vi "Move Parent FP to 0.vi"(8 "error in":errorcluster) -> (0 "error out":errorcluster)   [LabVIEW 2011]
doc: "Moves parent window to 0,0\n\n\nVersion 1.0 - 02/13/2013\n\nPhaeron, Inc.\nwww.phaeron.com\ninfo@phaeron.com"
uses:
  <vilib>/Utility/miscctls.llb/LVPointTypeDef.ctl
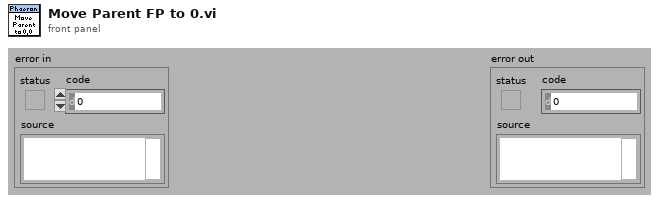
[diagram p1: front panel]
types:
  T1 = typedef "LVPointTypeDef.ctl" = cluster{"Horizontal":i16, "Vertical":i16}
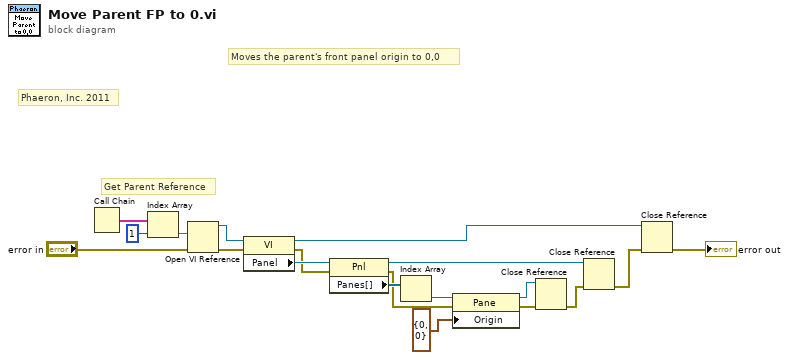
[diagram p0: block diagram]
diagram:
  # "Phaeron, Inc. 2011"
  # "Get Parent Reference"
  # "Moves the parent's front panel origin to 0,0"
  n1 = Call Chain() -> (call chain=w19:string[])
  n2 = Index Array(array=w19, index=1) -> (element=w17:string)
  n3 = Open VI Reference(vi path=w17, error in (no error)="error in") -> (vi reference=w16:refnum<vi>, error out=w9:errorcluster)  [unwired: 4 in]
  n4 = property class="VI"(reference=w16, error in=w9) -> (reference out=w2:refnum<vi>, error out=w14:errorcluster, "Panel"=w15:refnum<vi>)
  n5 = property class="Pnl"(reference=w15, error in=w14) -> (reference out=w4:refnum<vi>, error out=w10:errorcluster, "Panes[]"=w13:refnum<vi>[])
  n6 = Index Array(array=w13) -> (element=w12:refnum<vi>)  [unwired: 1 in]
  n7 = property class="Pane"(reference=w12, error in=w10, "Origin"=T1 {"Horizontal"=0, "Vertical"=0}) -> (reference out=w6:refnum<vi>, error out=w7:errorcluster)
  n8 = Close Reference(reference=w6, error in (no error)=w7) -> (error out=w5:errorcluster)
  n9 = Close Reference(reference=w4, error in (no error)=w5) -> (error out=w3:errorcluster)
  n10 = Close Reference(reference=w2, error in (no error)=w3) -> (error out=→"error out":errorcluster)
